vi "test Disconnect.vi"(8 "error in (no error)":errorcluster, 11 "TestCase in":refnum<class "Test Network Stream Transmission.lvclass">) -> (0 "error out":errorcluster, 3 "TestCase out":refnum<class "Test Network Stream Transmission.lvclass">)   [LabVIEW 2015]
uses:
  <vilib>/addons/_JKI Toolkits/VI Tester/TestCase.llb/TestCase.lvclass
  Test Network Stream Transmission.lvclass
  Protocols/Network Stream Strategy/Network Stream/Network Stream.lvclass
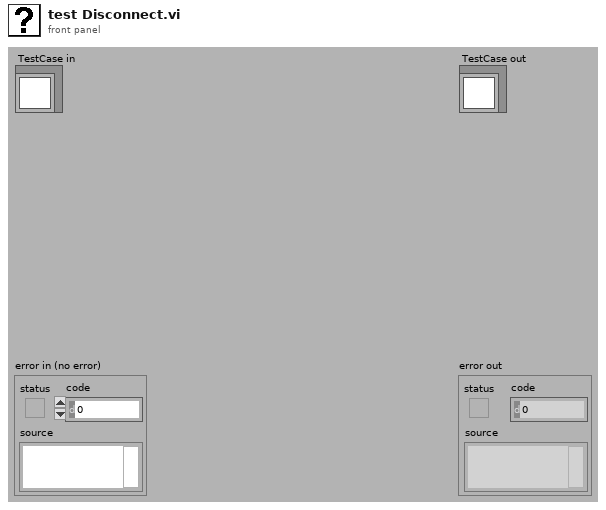
[diagram p1: front panel]
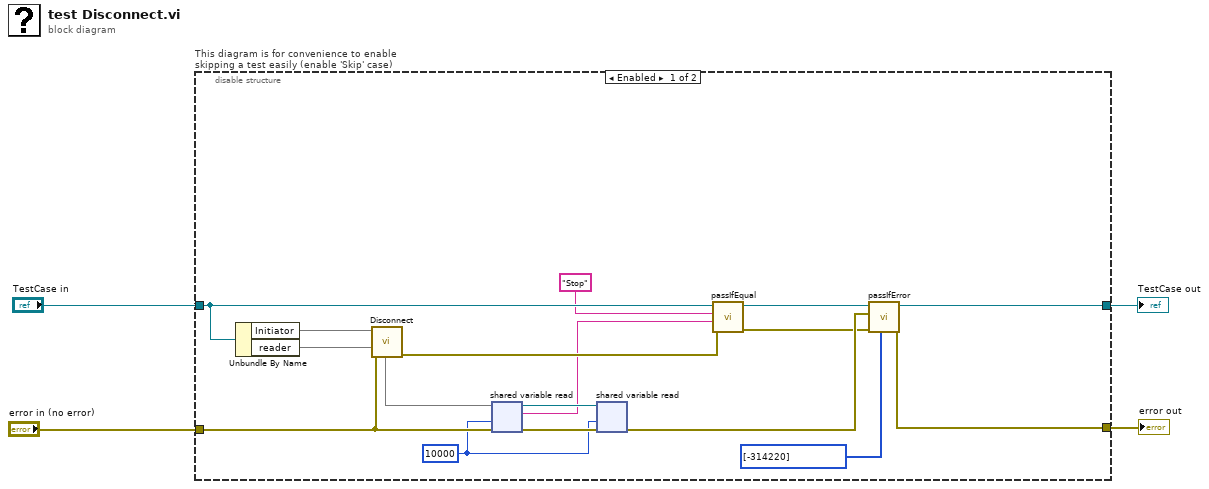
[diagram p0: block diagram]
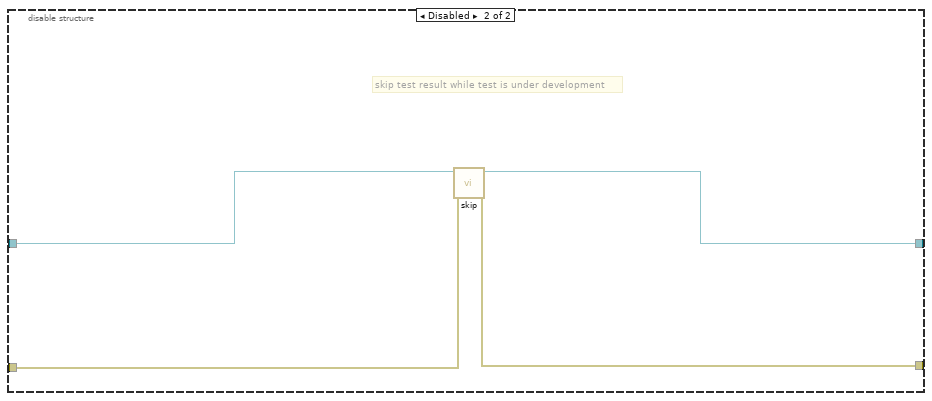
[diagram p2: hidden frame]
diagram:
  n1 = disable-structure "This diagram is for convenience to enable skipping a test easily (enable 'Skip' case)" shown="Enabled" {
    disable-tunnel: "TestCase in" -> [w12 w24]
    disable-tunnel: [w20 w22] -> w1
    disable-tunnel: [w19 w23] -> w3
    disable-tunnel: "error in (no error)" -> [w16 w21]
    frame Enabled {
      w5 = 10000 ("timeout ms (-1)")
      n2 = Unbundle By Name(w12) -> ("Initiator"=w18, "reader"=w17)
      n3 = call-dynamic "Disconnect.vi"("error in (no error)"=w16, "TCP Stream in"=w18) -> ("error out"=w8:errorcluster)  [unwired: 8 in, 1 out]
      n4 = shared-variable-read(w17, w16, w5) -> (w13:refnum<k21>, w14:errorcluster, w7:string)  [unwired: 1 out]
      n5 = shared-variable-read(w13, w14, w5) -> (w10:errorcluster)  [unwired: 3 out]
      n6 = call-dynamic "passIfEqual.vi"("error in (no error)"=w8, "y"=w7, "x"="Stop", "TestCase in"=w12) -> ("error out"=w9:errorcluster, "TestCase out"=w11:refnum<class "Test Network Stream Transmission.lvclass">)  [unwired: 6 in]
      n7 = call-dynamic "passIfError.vi"("passing error codes (default = any error code)"=i32[] [-314220], "error in (no error)"=w9, "error"=w10, "TestCase in"=w11) -> ("error out"=w19:errorcluster, "TestCase out"=w20:refnum<class "Test Network Stream Transmission.lvclass">)  [unwired: 6 in]
    }
    frame Disabled {
      # "skip test result while test is under development"
      n8 = call <vilib>:"skip.vi"("error in (no error)"=w21, "TestCase in"=w24) -> ("error out"=w23:errorcluster, "TestCase out"=w22:refnum<class "Test Network Stream Transmission.lvclass">)  [unwired: 8 in]
    }
  }
  "error out" <- w3
  "TestCase out" <- w1
